vi "Destructor.vi"(8 "error in":errorcluster, 11 "Document in":refnum<class "Characteristic.lvclass">) -> (0 "error out":errorcluster)   [LabVIEW 2021, in "ProligentXMLGenerator.lvlib" / "Characteristic.lvclass"]
uses:
  Characteristic.lvclass
  Characteristic.lvclass/Characteristic.ctl
  CustomData/CustomData.lvclass
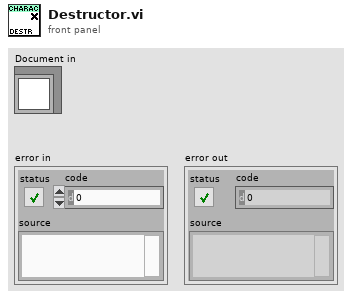
[diagram p1: front panel]
types:
  T1 = typedef "ProligentXMLGenerator.lvlib/Characteristic.lvclass/Data.ctl" = cluster{"Name":string, "CustomData":refnum<class "CustomData.lvclass">, "FullName":refnum<class "NonEmptyString_434.lvclass">, "Value":refnum<class "String_2000.lvclass">}
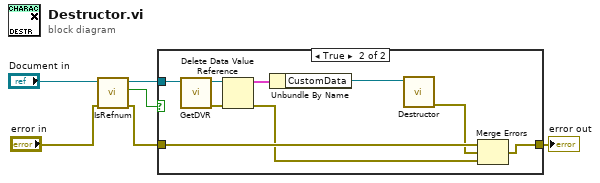
[diagram p0: block diagram]
diagram:
  n1 = call "IsRefnum.vi"("error in"="error in", "Document in"="Document in") -> ("error out"=w1:errorcluster, "IsRefnum"=w3:bool, "Document out"=w4:refnum<class "Characteristic.lvclass">)  [unwired: 7 in]
  n2 = case shown="True" w3 {
    tunnel: w1 -> [w7 w16]
    tunnel: [w7 w15] -> w6
    tunnel: w4 -> [_ w8]
    frame False {
    }
    frame True {
      n3 = call "GetDVR.vi"("Document in"=w8) -> ("error out"=w13:errorcluster, "DVRReference"=w14:refnum<data-value>)  [unwired: 9 in]
      n4 = Delete Data Value Reference(data value reference=w14, error in=w13) -> (data value=w11:T1, error out=w12:errorcluster)
      n5 = Unbundle By Name(w11) -> ("CustomData"=w10:refnum<class "CustomData.lvclass">)
      n6 = call "Destructor.vi"("CustomDataType"=w10) -> ("error out"=w9:errorcluster)  [unwired: 10 in]
      n7 = Merge Errors(w16, w9, w12) -> (w15:errorcluster)
    }
  }
  "error out" <- w6
